vi "HEWH Gas Thermal Final Calculations.vi"(0 "State5 Gal Water":dbl, 1 "State 5 Gal Gas":dbl, 2 "Thermal - Final Input":dbl[][](array[numeric]), 5 "Totalizer Gas":dbl, 7 "Mass Flow Gas":dbl, 9 "RTD Out (Deg F)":dbl, 11 "RTD In (Deg F)":dbl, 12 "Gallons (Gal)":dbl, 13 "Gross Heating Value, Vol (Real, Dry)":dbl) -> (3 "Thermal - Final Output":dbl[][](array[numeric]), 4 "Gas Totalizer Max":dbl, 6 "Mass Flow Avg":dbl format="%0.2f", 8 "RTD Out Avg":dbl format="%0.2f", 10 "RTD In Avg":dbl format="%0.2f", 14 "Heating Value Avg":dbl format="%0.2f", 15 "Gallons (Max)":dbl)   [LabVIEW 2023]
uses:
  <vilib>/Analysis/baseanly.llb/Mean (DBL).vi
  <vilib>/Analysis/NI_AALBase.lvlib
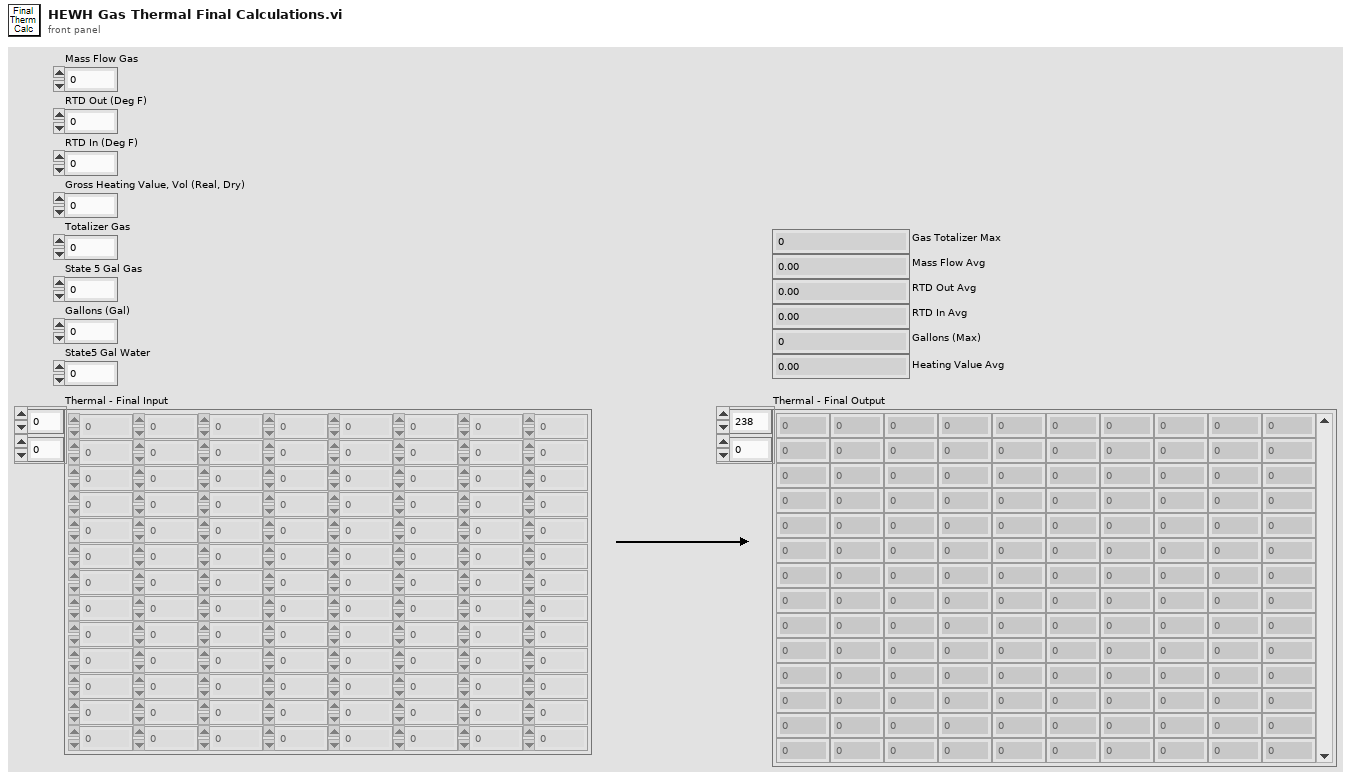
[diagram p1: front panel]
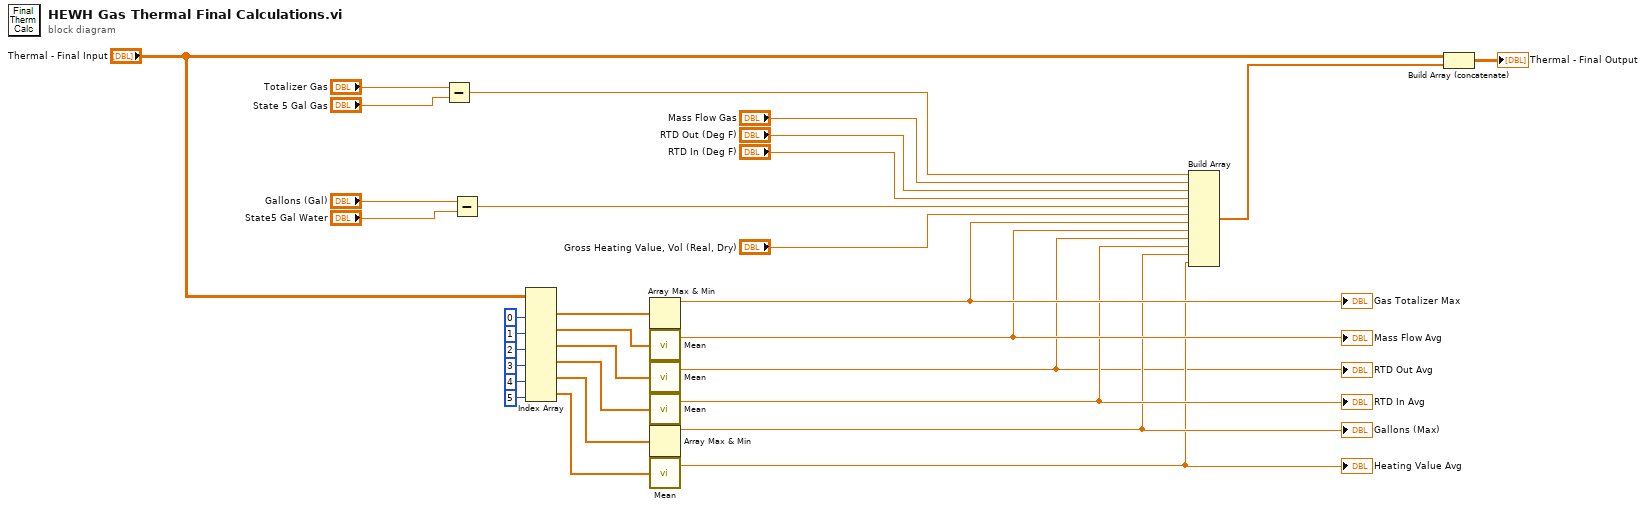
[diagram p0: block diagram]
diagram:
  n1 = Subtract(x="Totalizer Gas", y="State 5 Gal Gas") -> (x-y=w28:dbl)
  n2 = Subtract(x="Gallons (Gal)", y="State5 Gal Water") -> (x-y=w31:dbl)
  n3 = Index Array(array="Thermal - Final Input", index (col) #1=0 ("disabled index (col)"), index (col) #2=1 ("index (col)"), index (col) #3=2 ("index (col)"), index (col) #4=3 ("index (col)"), index (col) #5=4 ("index (col)"), index (col) #6=5 ("index (col)")) -> (element #1=w20:dbl[], element #2=w21:dbl[], element #3=w22:dbl[], element #4=w23:dbl[], element #5=w24:dbl[], element #6=w25:dbl[])  [unwired: 6 in]
  n4 = Array Max & Min(array=w20) -> (max value=w8:dbl)  [unwired: 3 out]
  "Gas Totalizer Max" <- w8
  n5 = call-poly <vilib>:"Mean.vi"("X"=w21) -> ("mean"=w7:dbl)  [unwired: 1 out]
  "Mass Flow Avg" <- w7
  n6 = call-poly <vilib>:"Mean.vi"("X"=w22) -> ("mean"=w3:dbl)  [unwired: 1 out]
  "RTD Out Avg" <- w3
  n7 = call-poly <vilib>:"Mean.vi"("X"=w23) -> ("mean"=w6:dbl)  [unwired: 1 out]
  "RTD In Avg" <- w6
  n8 = Array Max & Min(array=w24) -> (max value=w5:dbl)  [unwired: 3 out]
  "Gallons (Max)" <- w5
  n9 = call-poly <vilib>:"Mean.vi"("X"=w25) -> ("mean"=w4:dbl)  [unwired: 1 out]
  "Heating Value Avg" <- w4
  n10 = Build Array(w28, "Mass Flow Gas", "RTD Out (Deg F)", "RTD In (Deg F)", w31, "Gross Heating Value, Vol (Real, Dry)", w8, w7, w3, w6, w5, w4) -> (w13:dbl[])
  n11 = Build Array (concatenate)("Thermal - Final Input", w13) -> (→"Thermal - Final Output":dbl[][])
